vi "THzTime_SPEED_control_TA_170214.vi"(1 "ESP300 Axis":i8=1, 2 "ESP300 Address":string="1", 4 "Lockin Address":string="12") -> ()   [LabVIEW 2010]
panel:
  in  "Axis 2 Step btw Pos":dbl=1.0
  in  "Axis 1 Step btw Pos":dbl=1.0
  in  "Axis 2 # of Pos":u16=6
  in  "Delay":u32=10000
  in  "?":bool
  in  "# of Avg":i32=20
  in  "Axis 2 Starting Pos":dbl=-35.7
  in  "Axis 1 # of Pos":u16=6
  in  "Axis 1 Starting Pos":dbl=1.0
  in  "SHOT202 Address":string="8"
  out "Y position":dbl=-0.2690666666666667 format="%#.3p"
  out "X position":dbl=-0.49996666666666667 format="%#.3p"
  out "Power meter":dbl=48.71333333333333 format="%#.3p"
  in  "Save File Name":string="ref_sam_"
  in  "Launch server?":bool
  in  "Authorize?":bool=TRUE
  in  "CONEX-PSD9 Instrument Key 2":string="CONEX-PSD (A6ULD73M)"
  in  "Interdelay (ms)":dbl=20.0
  in  "pre delay(ms)":dbl=300.0
  out "Lock-in Y-Channel":dbl=3.63801e-12 format="%#.3p"
  out "Lock-in X-Channel":dbl=-3.4561e-11 format="%#.3p"
  out "THz Time-domain Signal Wave":cluster{"x-axis":sgl[], "y-axis":dbl[]}(graph)={"x-axis"=[-14.5, -14.51, -14.52, -14.53, -14.54, -14.55, -14.56, -14.57, -14.58, -14.59, -14.6, -14.61], "y-axis"=[1.819e-12, 1.819e-12, 0.0, 0.0, -1.819e-12, -7.27601e-12, -9.095e-12, -1.0914e-11, -1.6371e-11, -2.0009e-11, -2.1828e-11, -2.91041e-11]}
  in  "Autosave Directory for Long-term Average Scan":path=path "D:/taianh/Measurement Data/170202 Ref Sam"
  in  "OK Button":bool
  out "Data Type":string="outp ? 1"
  in  "Enum":enum16{"X", "Y", "Abs"}(ring)
  in  "Draw":bool
  in  "Exit Program":bool
  in  "Short term \nAverage#":i8=1
  in  "Step":sgl=0.005 min=0 max=10000 format="%.3f"
  in  "End Position":sgl=-18.0 min=-75 max=75 format="%#.3f"
  in  "Start Position":sgl=-14.5 min=-75 max=75 format="%#.3f"
  # "THz Experiment"
  # "Data"
  # "Auto-offset"
  # "Start Position (mm)"
  # "End Position (mm)"
  # "Step (mm)"
  # "Point Avg"
  # "# of Avg"
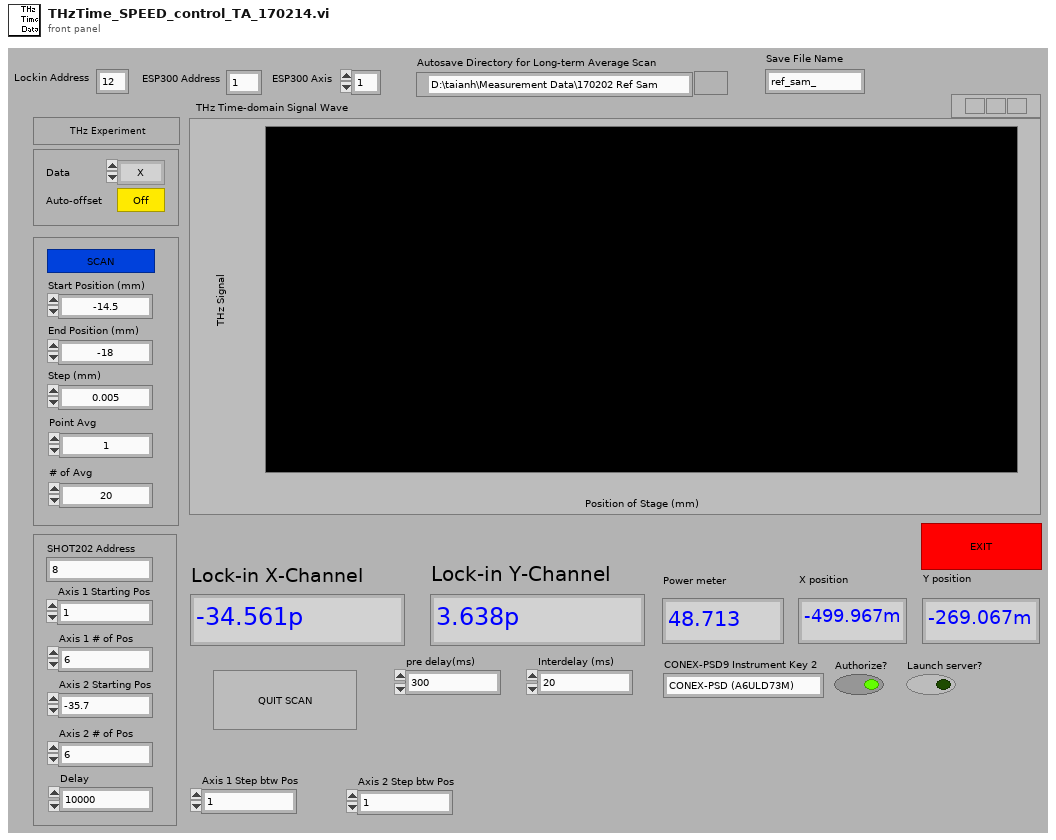
[diagram p1: front panel]
types:
  T1 = cluster{"ConexPSD Reference":refnum<k24>, "error out":errorcluster, "Component ID":i32}
  T2 = cluster{"Step Number":i32, "Step":sgl, "Start Position":sgl, "Time-out":i32, "Lockin Address":string, "Short term \nAverage#":i8, i32, "ESP300 Axis":i8, "Value":string, "pre delay(ms)":dbl, "Interdelay (ms)":dbl, "Autosave Directory for Long-term Average Scan":path, cluster{"ConexPSD Reference":refnum<k24>, "error out":errorcluster, "Component ID":i32}}
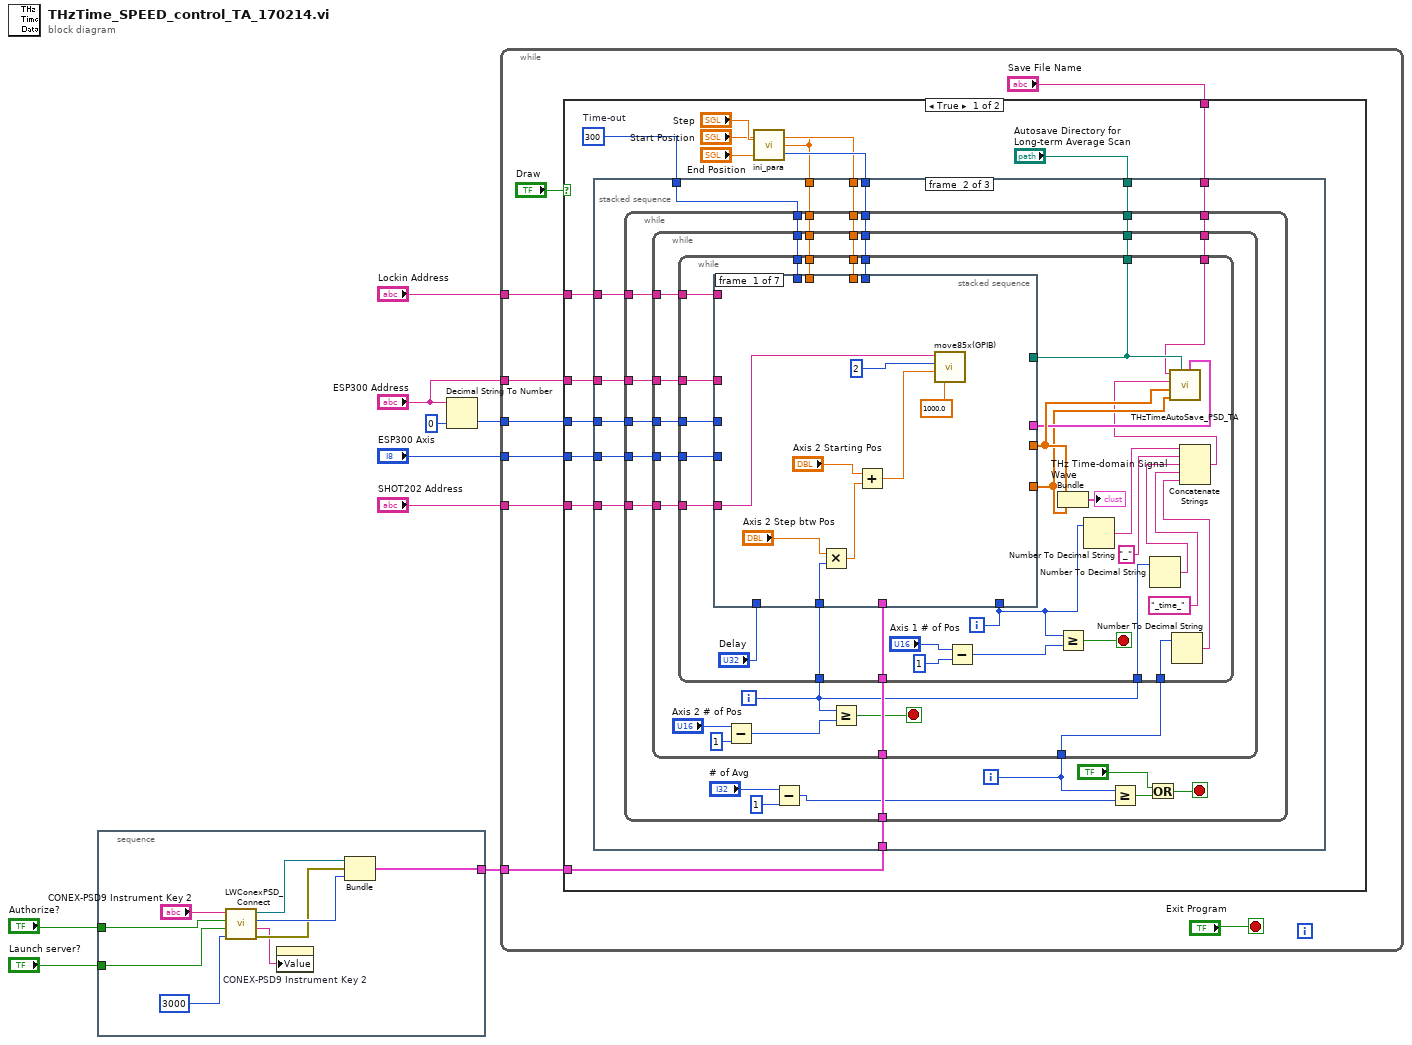
[diagram p0: block diagram]
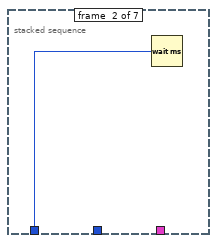
[diagram p3: hidden frame]
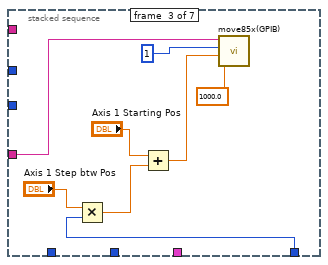
[diagram p4: hidden frame]
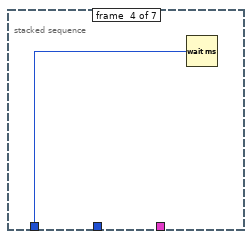
[diagram p5: hidden frame]
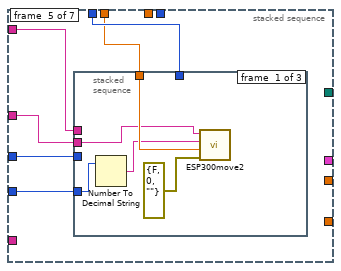
[diagram p6: hidden frame]
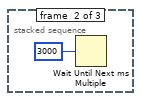
[diagram p7: hidden frame]
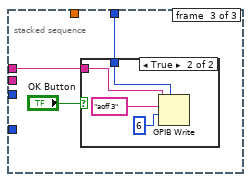
[diagram p8: hidden frame]
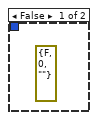
[diagram p9: hidden frame]
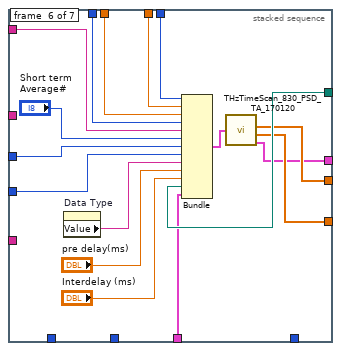
[diagram p10: hidden frame]
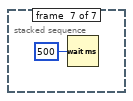
[diagram p11: hidden frame]
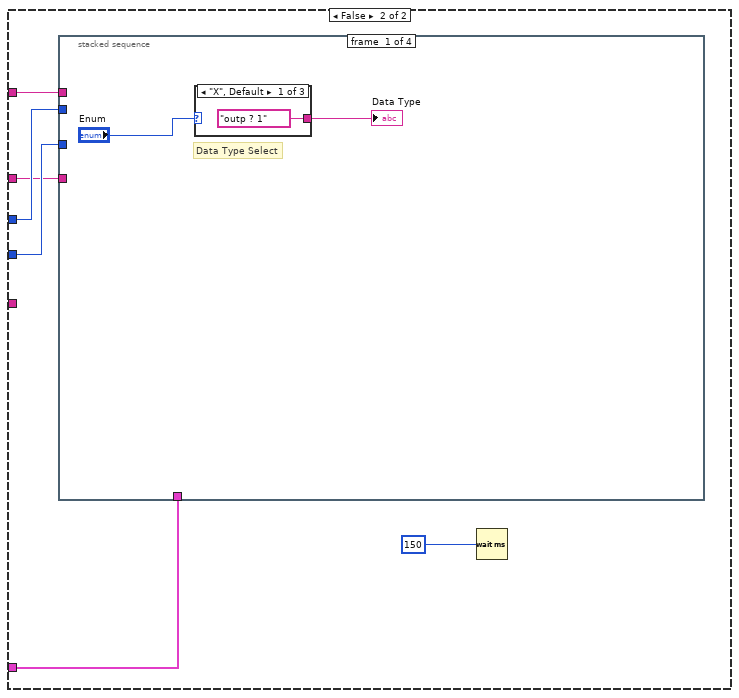
[diagram p13: hidden frame]
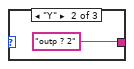
[diagram p14: hidden frame]
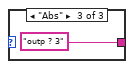
[diagram p15: hidden frame]
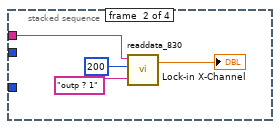
[diagram p16: hidden frame]
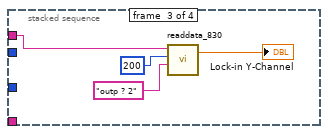
[diagram p17: hidden frame]
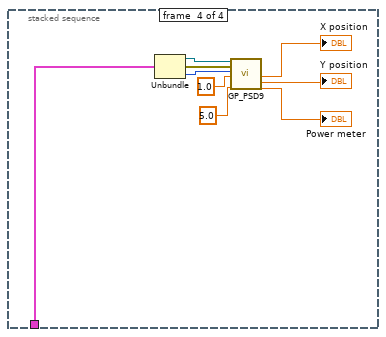
[diagram p18: hidden frame]
diagram:
  n1 = stacked-sequence {
    tunnel: "Authorize?" -> [w12]
    tunnel: [w11] -> w2
    tunnel: "Launch server?" -> [w10]
    frame #0 {
      n2 = call "LWConexPSD_Connect.vi"("DiscoverTimeout (10000 msec)"=3000, "Launch server? (True)"=w10, "Authorize? (True)"=w12, "Instrument Key"="CONEX-PSD9 Instrument Key 2") -> ("error out"=w16:errorcluster, "Instrument Key out"=w14:string, "Component ID"=w17:i32, "ConexPSD Reference"=w15:refnum<k24>)
      n3 = property on="CONEX-PSD9 Instrument Key 2" class="Str"("Value"=w14) -> ()  [unwired: 2 in, 2 out]
      n4 = Bundle("ConexPSD Reference"=w15, "error out"=w16, "Component ID"=w17) -> (w11:T1)  [unwired: 1 in]
    }
  }
  n5 = Decimal String To Number(string="ESP300 Address", default (0L)=0 ("default (0 I32)")) -> (number=w7:i32)  [unwired: 1 in, 1 out]
  n6 = while {
    tunnel: "ESP300 Axis" -> [w25]
    tunnel: "Lockin Address" -> [w24]
    tunnel: w7 -> [w23]
    tunnel: "ESP300 Address" -> [w22]
    tunnel: w2 -> [w21]
    tunnel: "SHOT202 Address" -> [w19]
    stop <- "Exit Program" stop-if-true
    n7 = case shown="True" "Draw" {
      tunnel: w24 -> [w41 w180]
      tunnel: w25 -> [w40 w182]
      tunnel: w23 -> [w39 w181]
      tunnel: w22 -> [w31 w178]
      tunnel: w21 -> [w30 w177]
      tunnel: "Save File Name" -> [w29 _]
      tunnel: w19 -> [w28 _]
      frame True {
        w38 = 300  # Time-out
        n8 = call "ini_para.vi"("End Position"="End Position", "Start Position"="Start Position", "Step"="Step") -> ("Step Number"=w35:i32, "Step"=w34:sgl)
        n9 = stacked-sequence {
          tunnel: w41 -> [_ w53 _]
          tunnel: w38 -> [_ w52 _]
          tunnel: w40 -> [_ w51 _]
          tunnel: w39 -> [_ w50 _]
          tunnel: w35 -> [_ w48 _]
          tunnel: w34 -> [_ w46 _]
          tunnel: "Start Position" -> [_ w49 _]
          tunnel: "Autosave Directory for Long-term Average Scan" -> [_ w47 _]
          tunnel: w31 -> [_ w45 _]
          tunnel: w30 -> [_ w44 _]
          tunnel: w29 -> [_ w43 _]
          tunnel: w28 -> [_ w42 _]
          frame #0 {
          }
          frame #1 {
            n10 = while {
              tunnel: w53 -> [w72]
              tunnel: w52 -> [w71]
              tunnel: w51 -> [w70]
              tunnel: w50 -> [w69]
              tunnel: w49 -> [w68]
              tunnel: w48 -> [w67]
              tunnel: w47 -> [w66]
              tunnel: w46 -> [w65]
              tunnel: w45 -> [w64]
              tunnel: w44 -> [w63]
              tunnel: w43 -> [w62]
              tunnel: w42 -> [w61]
              i -> [w54]
              stop <- w56 stop-if-true
              n11 = while {
                tunnel: w72 -> [w90]
                tunnel: w71 -> [w89]
                tunnel: w70 -> [w88]
                tunnel: w69 -> [w87]
                tunnel: w68 -> [w86]
                tunnel: w67 -> [w85]
                tunnel: w66 -> [w84]
                tunnel: w65 -> [w83]
                tunnel: w64 -> [w82]
                tunnel: w63 -> [w81]
                tunnel: w62 -> [w80]
                tunnel: w61 -> [w79]
                tunnel: w54 -> [w73]
                i -> [w74]
                stop <- w78 stop-if-true
                n12 = while {
                  tunnel: w89 -> [w120]
                  tunnel: w90 -> [w121]
                  tunnel: w88 -> [w119]
                  tunnel: w87 -> [w118]
                  tunnel: w86 -> [w117]
                  tunnel: w83 -> [w116]
                  tunnel: w85 -> [w115]
                  tunnel: w84 -> [w110]
                  tunnel: w82 -> [w113]
                  tunnel: w81 -> [w112]
                  tunnel: w80 -> [w109]
                  tunnel: w79 -> [w106]
                  tunnel: w74 -> [w103]
                  tunnel: w74 -> [w98]
                  tunnel: w73 -> [w92]
                  i -> [w99]
                  stop <- w105 stop-if-true
                  n13 = stacked-sequence {
                    tunnel: w121 -> [_ _ _ _ w145 w171 _]
                    tunnel: w120 -> [_ _ _ _ w144 w172 _]
                    tunnel: w119 -> [_ _ _ _ w143 w168 _]
                    tunnel: w118 -> [_ _ _ _ w142 w169 _]
                    tunnel: w117 -> [_ _ _ _ w141 w173 _]
                    tunnel: w116 -> [_ _ _ _ _ w174 _]
                    tunnel: w115 -> [_ _ _ _ _ w175 _]
                    tunnel: [_ _ _ _ _ w162 _] -> w111
                    tunnel: [_ _ _ _ _ w161 _] -> w107
                    tunnel: w113 -> [_ _ _ _ w140 _ _]
                    tunnel: w110 -> [_ _ _ _ _ w164 _]
                    tunnel: w112 -> [_ _ _ _ _ w163 _]
                    tunnel: [_ _ _ _ _ w160 _] -> w108
                    tunnel: w106 -> [w129 _ w138 _ _ _ _]
                    tunnel: w99 -> [_ _ w136 _ _ _ _]
                    tunnel: "Delay" -> [_ w130 _ w139 _ _ _]
                    tunnel: w103 -> [w127 _ _ _ _ _ _]
                    frame #0 {
                      n14 = Multiply(x="Axis 2 Step btw Pos", y=w127) -> (x*y=w125:dbl)
                      n15 = Add(x="Axis 2 Starting Pos", y=w125) -> (x+y=w124:dbl)
                      n16 = call "move85x(GPIB).vi"("wait time(ms)"=1000.0, "Moving Distance (mm) : resolutino is 1um"=w124, "Axis Number"=u8 2, "SHOT202 Address"=w129) -> ()
                    }
                    frame #1 {
                      n17 = Wait (ms)(milliseconds to wait=w130) -> ()  [unwired: 1 out]
                    }
                    frame #2 {
                      n18 = Multiply(x="Axis 1 Step btw Pos", y=w136) -> (x*y=w133:dbl)
                      n19 = Add(x="Axis 1 Starting Pos", y=w133) -> (x+y=w132:dbl)
                      n20 = call "move85x(GPIB).vi"("wait time(ms)"=1000.0, "Moving Distance (mm) : resolutino is 1um"=w132, "Axis Number"=u8 1, "SHOT202 Address"=w138) -> ()
                    }
                    frame #3 {
                      n21 = Wait (ms)(milliseconds to wait=w139) -> ()  [unwired: 1 out]
                    }
                    frame #4 {
                      n22 = stacked-sequence {
                        tunnel: w145 -> [_ _ w153]
                        tunnel: w144 -> [_ _ w152]
                        tunnel: w143 -> [w147 _ _]
                        tunnel: w142 -> [_ _ _]
                        tunnel: w141 -> [w150 _ _]
                        tunnel: w140 -> [w148 _ _]
                        frame #0 {
                          n23 = Number To Decimal String(number=w147) -> (decimal integer string=w146:string)  [unwired: 1 in]
                          n24 = call "ESP300move2.vi"("ESP300 Address"=w148, "ESP300 Channel"=w146, "Target"=w150, "error in (no error) 2"=errorcluster {"status"=FALSE, "code"=0, "source"=""}) -> ()  [unwired: 6 in, 1 out]
                        }
                        frame #1 {
                          n25 = Wait Until Next ms Multiple(millisecond multiple=3000) -> ()  [unwired: 1 out]
                        }
                        frame #2 {
                          n26 = case shown="True" "OK Button" {
                            tunnel: w153 -> [_ w158]
                            tunnel: w152 -> [_ w156]
                            frame False {
                              (unwired) errorcluster {"status"=FALSE, "code"=0, "source"=""} ("error in")
                            }
                            frame True {
                              n27 = GPIB Write(0:w158, 1:"aoff 3" ("data"), 2:i16 6 ("mode (0)"), 4:w156) -> ()  [unwired: 1 in, 2 out]
                            }
                          }
                        }
                      }
                    }
                    frame #5 {
                      n28 = property on="Data Type" class="Str"() -> ("Value"=w167:string)  [unwired: 2 in, 2 out]
                      n29 = Bundle("Step Number"=w175, "Step"=w174, "Start Position"=w173, "Time-out"=w172, "Lockin Address"=w171, "Short term \nAverage#"="Short term \nAverage#", w169, "ESP300 Axis"=w168, "Value"=w167, "pre delay(ms)"="pre delay(ms)", "Interdelay (ms)"="Interdelay (ms)", "Autosave Directory for Long-term Average Scan"=w164, w163) -> (w159:T2)  [unwired: 1 in]
                      n30 = call "THzTimeScan_830_PSD_TA_170120.vi"("input"=w159) -> ("x-axis"=w162:sgl[], "y-axis"=w161:dbl[], "ext. out"=w160:cluster{dbl[], dbl[], dbl[], dbl[], string[]})  [unwired: 1 out]
                    }
                    frame #6 {
                      n31 = Wait (ms)(milliseconds to wait=u32 500) -> ()  [unwired: 1 out]
                    }
                  }
                  n32 = Subtract(x="Axis 1 # of Pos", y=u16 1) -> (x-y=w100:u16)
                  n33 = Bundle("x-axis"=w111, "y-axis"=w107) -> (→"THz Time-domain Signal Wave":cluster{"x-axis":sgl[], "y-axis":dbl[]})  [unwired: 1 in]
                  n34 = Greater Or Equal?(x=w99, y=w100) -> (x >= y?=w105:bool)
                  n35 = Number To Decimal String(number=w99) -> (decimal integer string=w97:string)  [unwired: 1 in]
                  n36 = Number To Decimal String(number=w98) -> (decimal integer string=w94:string)  [unwired: 1 in]
                  n37 = Number To Decimal String(number=w92) -> (decimal integer string=w91:string)  [unwired: 1 in]
                  n38 = Concatenate Strings(w97, "_", w94, "_time_", w91) -> (w95:string)
                  n39 = call "THzTimeAutoSave_PSD_TA.vi"("ext. out"=w108, "Autosave Directory for Long-term Average Scan"=w110, "y-axis"=w107, "x-axis"=w111, "String"=w95, "SaveFile name"=w109) -> ()  [unwired: 4 in]
                }
                n40 = Subtract(x="Axis 2 # of Pos", y=u16 1) -> (x-y=w75:u16)
                n41 = Greater Or Equal?(x=w74, y=w75) -> (x >= y?=w78:bool)
              }
              n42 = Subtract(x="# of Avg", y=1) -> (x-y=w55:i32)
              n43 = Greater Or Equal?(x=w54, y=w55) -> (x >= y?=w58:bool)
              n44 = Or(x="?", y=w58) -> (x .or. y?=w56:bool)
            }
          }
          frame #2 {
          }
        }
      }
      frame False {
        n45 = stacked-sequence {
          tunnel: w182 -> [_ _ _ _]
          tunnel: w181 -> [_ _ _ _]
          tunnel: w180 -> [_ w191 w195 _]
          tunnel: w178 -> [_ _ _ _]
          tunnel: w177 -> [_ _ _ w196]
          frame #0 {
            # "Data Type Select"
            n46 = case shown="\"X\", Default" "Enum" {
              tunnel: ["outp ? 1" "outp ? 2" "outp ? 3"] -> w184
              frame "X", Default {
              }
              frame "Y" {
              }
              frame "Abs" {
              }
            }
            "Data Type" <- w184
          }
          frame #1 {
            n47 = call "readdata_830.vi"("Command"="outp ? 1", "timeout"=200, "Lockin Address"=w191) -> ("Data"=→"Lock-in X-Channel":dbl)  [unwired: 1 in, 1 out]
          }
          frame #2 {
            n48 = call "readdata_830.vi"("Command"="outp ? 2", "timeout"=200, "Lockin Address"=w195) -> ("Data"=→"Lock-in Y-Channel":dbl)  [unwired: 1 in, 1 out]
          }
          frame #3 {
            n49 = Unbundle(w196) -> ("ConexPSD Reference"=w204:refnum<k24>, "error out"=w203:errorcluster, "Component ID"=w202:i32)
            n50 = call "GP_PSD9.vi"("ConexPSD Reference"=w204, "error out"=w203, "Component ID"=w202, "Adress"=1.0 ("shot average"), "shot average"=5.0) -> ("PositionX"=→"X position":dbl, "PositionY"=→"Y position":dbl, "LaserPower"=→"Power meter":dbl)  [unwired: 8 in, 4 out]
          }
        }
        n51 = Wait (ms)(milliseconds to wait=u32 150) -> ()  [unwired: 1 out]
      }
    }
  }
